vi "HJ212-2017.vi"(8 "error in (no error)":errorcluster caption="错误输入（无错误）", 10 "PWD？":bool, 11 "数据段":T1) -> (0 "error out":errorcluster caption="错误输出", 2 "通讯包字符串":string, 3 "通讯包":T2={"包头（2）"="##", "数据段长度（4）"="", "数据段"="", "CRC校验"="", "包尾"=""})   [LabVIEW 2016, in "数据传输系统.lvlib"]
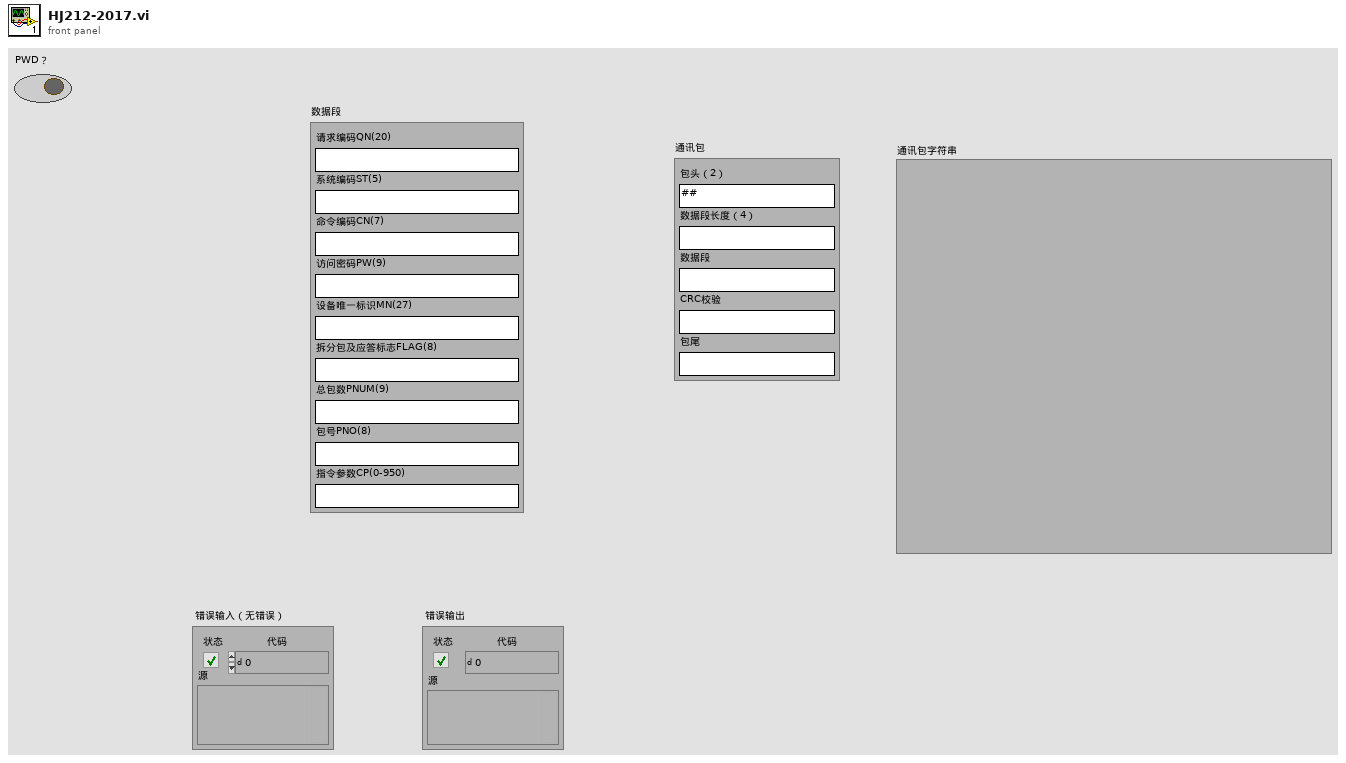
[diagram p1: front panel]
types:
  T1 = cluster{"请求编码QN(20)":string, "系统编码ST(5)":string, "命令编码CN(7)":string, "访问密码PW(9)":string, "设备唯一标识MN(27)":string, "拆分包及应答标志FLAG(8)":string, "总包数PNUM(9)":string, "包号PNO(8)":string, "指令参数CP(0-950)":string}
  T2 = cluster{"包头（2）":string, "数据段长度（4）":string, "数据段":string, "CRC校验":string, "包尾":string}
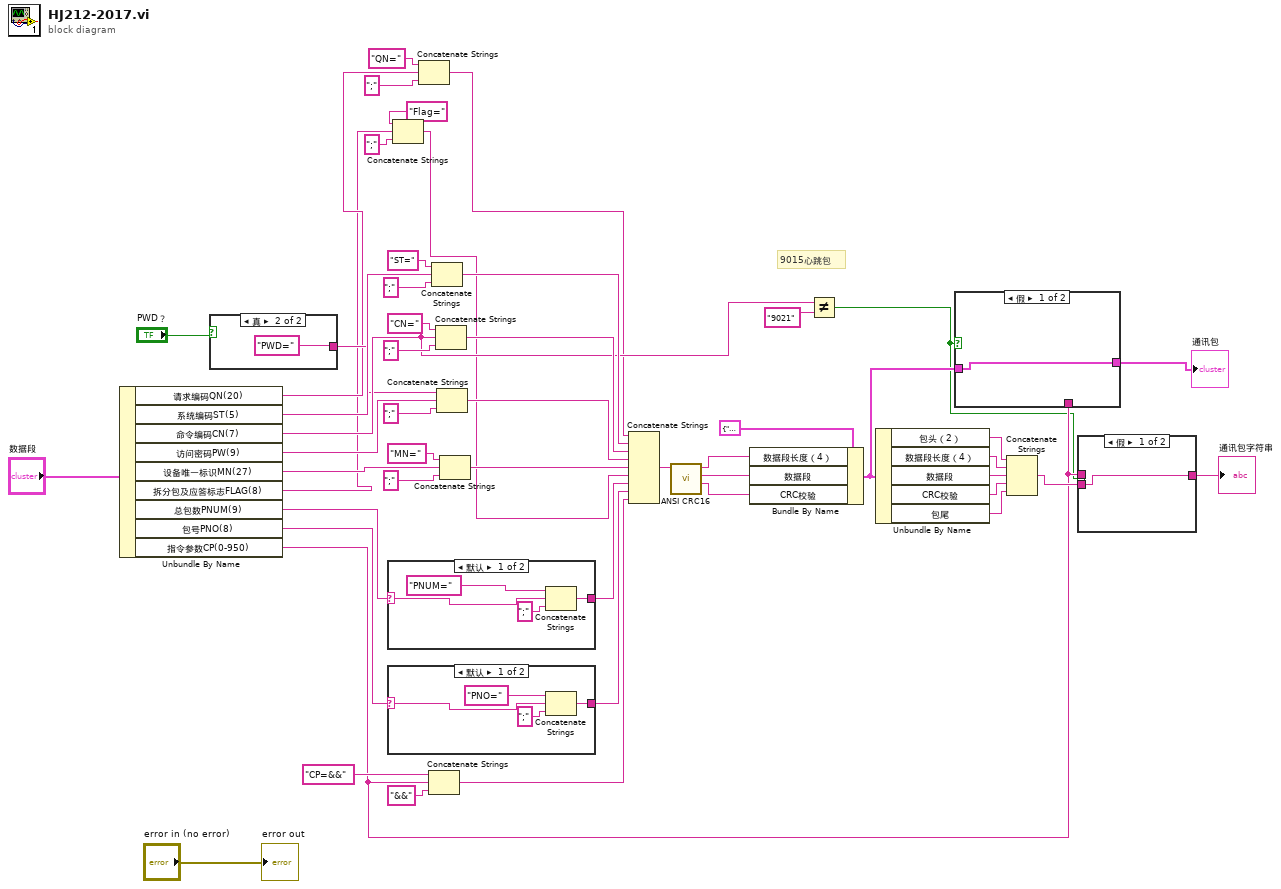
[diagram p0: block diagram]
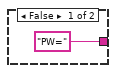
[diagram p2: hidden frame]
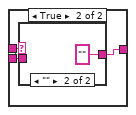
[diagram p3: hidden frame]
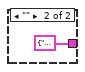
[diagram p6: hidden frame]
diagram:
  # "9015心跳包"
  n1 = Unbundle By Name("数据段") -> ("请求编码QN(20)"=w8:string, "系统编码ST(5)"=w50:string, "命令编码CN(7)"=w13:string, "访问密码PW(9)"=w46:string, "设备唯一标识MN(27)"=w44:string, "拆分包及应答标志FLAG(8)"=w6:string, "总包数PNUM(9)"=w36:string, "包号PNO(8)"=w34:string, "指令参数CP(0-950)"=w14:string)
  n2 = case shown="真" "PWD？" {
    tunnel: ["PW=" ("字符串") "PWD=" ("字符串")] -> w9
    frame False {
    }
    frame True {
    }
  }
  n3 = case shown="默认" w36 {
    selector: w36 -> [w56 w58]
    tunnel: [w54 w58] -> w35
    frame Default {
      n4 = Concatenate Strings("PNUM=" ("字符串"), w56, ";" ("字符串")) -> (w54:string)
    }
    frame "" {
    }
  }
  n5 = case shown="默认" w34 {
    selector: w34 -> [w61 w63]
    tunnel: [w59 w63] -> w33
    frame Default {
      n6 = Concatenate Strings("PNO=" ("字符串"), w61, ";" ("字符串")) -> (w59:string)
    }
    frame "" {
    }
  }
  n7 = Concatenate Strings("Flag=" ("字符串"), w6, ";" ("字符串")) -> (w5:string)
  n8 = Concatenate Strings("QN=" ("字符串"), w8, ";" ("字符串")) -> (w7:string)
  n9 = Concatenate Strings("CP=&&" ("字符串"), w14, "&&" ("字符串")) -> (w30:string)
  n10 = Concatenate Strings("ST=" ("字符串"), w50, ";" ("字符串")) -> (w41:string)
  n11 = Concatenate Strings("CN=" ("字符串"), w13, ";" ("字符串")) -> (w40:string)
  n12 = Concatenate Strings(w9, w46, ";" ("字符串")) -> (w39:string)
  n13 = Concatenate Strings("MN=" ("字符串"), w44, ";" ("字符串")) -> (w38:string)
  n14 = Concatenate Strings(w7, w41, w40, w39, w38, w5, w35, w33, w30) -> (w29:string)
  n15 = call "ANSI CRC16.vi"("puchMsg"=w29) -> ("CRC校验"=w19:string, "数据段"=w20:string, "数据段长度"=w21:string)  [unwired: 8 in]
  n16 = Bundle By Name(cluster=T2 {"包头（2）"="##", "数据段长度（4）"="", "数据段"="", "CRC校验"="", "包尾"="\r\n"} ("通讯包"), "数据段长度（4）"=w21, "数据段"=w20, "CRC校验"=w19) -> (w16:T2)
  n17 = Not Equal?(x=w13, y="9021") -> (x != y?=w11:bool)
  n18 = Unbundle By Name(w16) -> ("包头（2）"=w26:string, "数据段长度（4）"=w25:string, "数据段"=w24:string, "CRC校验"=w23:string, "包尾"=w22:string)
  n19 = case shown="假" w11 {
    tunnel: w16 -> [w64 w67]
    tunnel: [w64 w66] -> w15
    tunnel: w14 -> [_ w65]
    frame False {
    }
    frame True {
      n20 = case shown="\"假\", 默认" w65 {
        tunnel: [w68 T2 {"包头（2）"="", "数据段长度（4）"="", "数据段"="", "CRC校验"="", "包尾"=""} ("通讯包")] -> w66
        tunnel: w67 -> [w68 _]
        frame "假", Default {
        }
        frame "" {
        }
      }
    }
  }
  "通讯包" <- w15
  n21 = Concatenate Strings(w26, w25, w24, w23, w22) -> (w18:string)
  n22 = case shown="假" w11 {
    tunnel: w18 -> [w70 w73]
    tunnel: [w70 w72] -> w17
    tunnel: w14 -> [_ w71]
    frame False {
    }
    frame True {
      n23 = case shown="\"\"" w71 {
        tunnel: [w74 ""] -> w72
        tunnel: w73 -> [w74 _]
        frame "假", Default {
        }
        frame "" {
        }
      }
    }
  }
  "通讯包字符串" <- w17
  "error out" <- "error in (no error)"
